vi "BrowerFactory.vi"(8 "error in (no error)":errorcluster, 10 "BrowerIndex(0)":i32, 11 "AbstractBuilder in":refnum<class "AbstractBuilder.lvclass">) -> (0 "error out":errorcluster, 2 "BrowerComponent":refnum<class "BrowerComponent.lvclass">, 3 "AbstractBuilder out":refnum<class "AbstractBuilder.lvclass">)   [LabVIEW 2015, in "AbstractBuilder.lvclass"]
uses:
  AbstractBuilder.lvclass
  BrowerComponent/BrowerComponent/BrowerComponent.lvclass
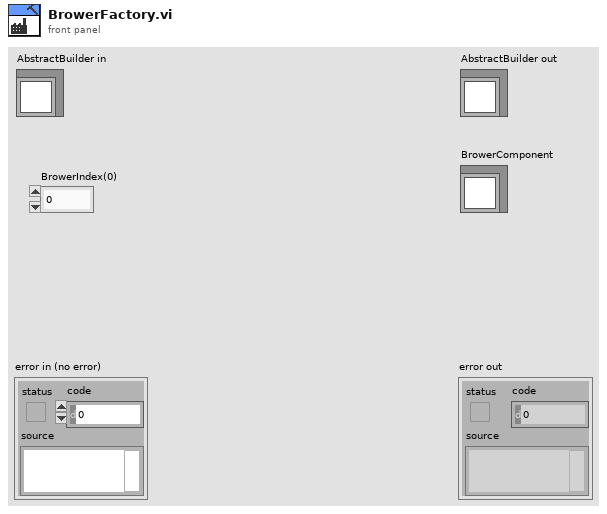
[diagram p1: front panel]
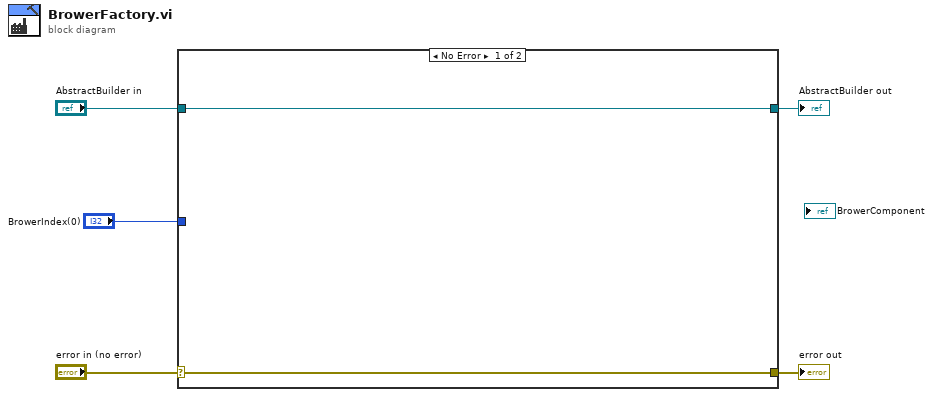
[diagram p0: block diagram]
diagram:
  n1 = case shown="No Error" "error in (no error)" {
    selector: "error in (no error)" -> [w6 w9]
    tunnel: [w6 w9] -> w4
    tunnel: [w7 w8] -> w2
    tunnel: "AbstractBuilder in" -> [w7 w8]
    tunnel: "BrowerIndex(0)" -> [_ _]
    frame No Error {
    }
    frame Error {
    }
  }
  "error out" <- w4
  "AbstractBuilder out" <- w2
